vi "Main.vi"() -> ()   [LabVIEW 2019]
uses:
  Controls/States.ctl
  <vilib>/Gustavo Trejo/PIC Serial Toolkit/Controls/TRISA.ctl
  <vilib>/Gustavo Trejo/PIC Serial Toolkit/Controls/TRISB.ctl
  <vilib>/Gustavo Trejo/PIC Serial Toolkit/Controls/TRISC.ctl
  <vilib>/Gustavo Trejo/PIC Serial Toolkit/Controls/TRISD.ctl
  <vilib>/Gustavo Trejo/PIC Serial Toolkit/Controls/TRISE.ctl
  <vilib>/Gustavo Trejo/PIC Serial Toolkit/Controls/Pin Number.ctl
panel:
  out "Down":bool
  out "Up":bool
  in  "COM":refnum<visa-resource-name>
  out "Estado":string
  in  "Stop":bool
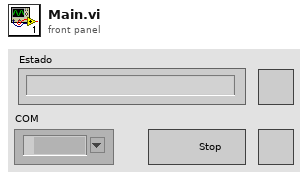
[diagram p1: front panel]
types:
  T1 = typedef "TRISE.ctl" = cluster{"E0":bool, "E1":bool, "E2":bool}
  T2 = typedef "TRISD.ctl" = cluster{"D0":bool, "D1":bool, "D2":bool, "D3":bool, "D4":bool, "D5":bool, "D6":bool, "D7":bool}
  T3 = typedef "TRISC.ctl" = cluster{"C0":bool, "C1":bool, "C2":bool, "C3":bool, "C4":bool, "C5":bool}
  T4 = typedef "TRISB.ctl" = cluster{"B0":bool, "B1":bool, "B2":bool, "B3":bool, "B4":bool, "B5":bool, "B6":bool, "B7":bool}
  T5 = typedef "TRISA.ctl" = cluster{"A0":bool, "A1":bool, "A2":bool, "A3":bool, "A4":bool, "A5":bool, "A6":bool, "A7":bool}
  T6 = typedef "States.ctl" = enum16{"Start", "GoDown", "BeDown", "GoUp", "BeUp", "Error", "Finish"}
  T7 = typedef "Pin Number.ctl" = enum16{"A0/AN0", "A1/AN1", "A2/AN2", "A3/AN3", "A4", "A5/AN4", "A6", "A7", "B0/AN12", "B1/AN10", "B2/AN8", "B3/AN9", "B4/AN11", "B5/AN13", "B6", "B7", "C0", "C1/PWM2", "C2/PWM1", "C3", "C4", "C5", "D0", "D1", "D2", "D3", "D4", "D5", "D6", "D7", "E0/AN5", "E1/AN6", "E2/AN7"}
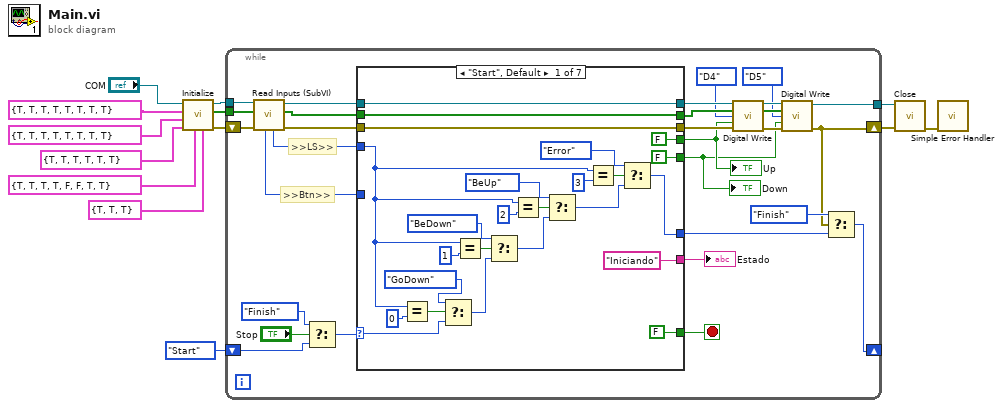
[diagram p0: block diagram]
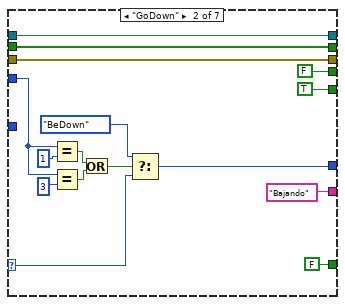
[diagram p2: hidden frame]
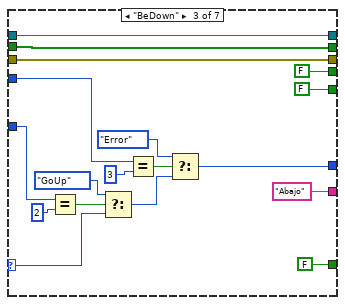
[diagram p3: hidden frame]
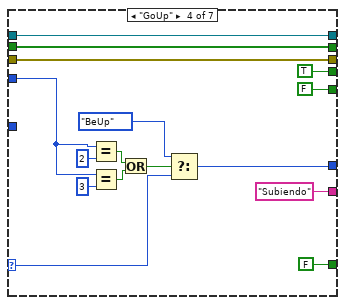
[diagram p4: hidden frame]
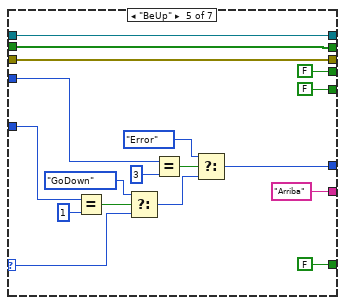
[diagram p5: hidden frame]
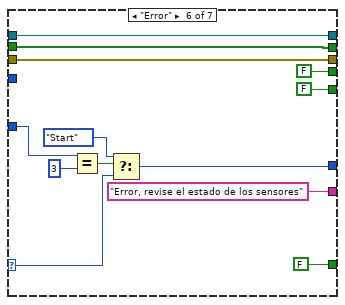
[diagram p6: hidden frame]
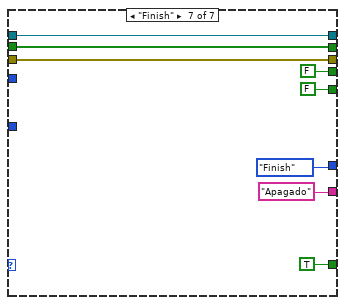
[diagram p7: hidden frame]
diagram:
  n1 = call <vilib>:"Initialize.vi"("TRISE E0-E2"=T1 {"E0"=TRUE, "E1"=TRUE, "E2"=TRUE}, "TRISD D0-D7"=T2 {"D0"=TRUE, "D1"=TRUE, "D2"=TRUE, "D3"=TRUE, "D4"=FALSE, "D5"=FALSE, "D6"=TRUE, "D7"=TRUE}, "TRISC C0-C5"=T3 {"C0"=TRUE, "C1"=TRUE, "C2"=TRUE, "C3"=TRUE, "C4"=TRUE, "C5"=TRUE}, "TRISB B0-B7"=T4 {"B0"=TRUE, "B1"=TRUE, "B2"=TRUE, "B3"=TRUE, "B4"=TRUE, "B5"=TRUE, "B6"=TRUE, "B7"=TRUE}, "TRISA A0-A7"=T5 {"A0"=TRUE, "A1"=TRUE, "A2"=TRUE, "A3"=TRUE, "A4"=TRUE, "A5"=TRUE, "A6"=TRUE, "A7"=TRUE}, "VISA Refnum in"="COM") -> ("error out"=w12:errorcluster, "Ports Ref Out"=w5:bool[], "VISA Refnum out"=w4:refnum<visa-resource-name>)  [unwired: 3 in]
  n2 = while {
    shift-right: [w36] -> _
    shift-left: States."Start" -> [w39]
    shift-right: [w16] -> w3
    shift-left: w12 -> [w33]
    tunnel: w5 -> [w31]
    tunnel: w4 -> [w30]
    tunnel: [w17] -> w2
    stop <- w38 stop-if-true
    # ">>LS>>"
    # ">>Btn>>"
    n3 = call "Read Inputs (SubVI).vi"("error in (no error)"=w33, "Ports Ref In"=w31, "VISA Refnum in"=w30) -> ("error out"=w32:errorcluster, "Ports Ref Out"=w26:bool[], "VISA Refnum out"=w27:refnum<visa-resource-name>, "LS"=w29:u32, "Btn"=w28:u32)  [unwired: 4 in]
    n4 = Select(t=States."Finish", s="Stop", f=w39) -> (s? t:f=w40:T6)
    n5 = case shown="\"Start\", Default" w40 {
      selector: w40 -> [w50 w77 w99 w103 w119 w137 _]
      tunnel: [FALSE FALSE FALSE FALSE FALSE FALSE TRUE] -> w38
      tunnel: [w66 w74 w90 w109 w125 w144 w154] -> w23
      tunnel: w32 -> [w66 w74 w90 w109 w125 w144 w154]
      tunnel: w29 -> [w52 w81 w96 w111 w127 _ _]
      tunnel: w28 -> [_ _ w101 _ w128 w148 _]
      tunnel: [w51 w75 w91 w110 w126 w138 States."Finish"] -> w35
      tunnel: ["Iniciando" "Bajando" "Abajo" "Subiendo" "Arriba" "Error, revise el estado de los sensores" "Apagado"] -> w34
      tunnel: [FALSE ("Abajo") TRUE ("Abajo") FALSE ("Abajo") FALSE ("Abajo") FALSE ("Abajo") FALSE ("Abajo") FALSE ("Abajo")] -> w14
      tunnel: [FALSE ("Arriba") FALSE ("Arriba") FALSE ("Arriba") TRUE ("Arriba") FALSE ("Arriba") FALSE ("Arriba") FALSE ("Arriba")] -> w15
      tunnel: [w44 w69 w85 w104 w120 w139 w150] -> w25
      tunnel: w27 -> [w44 w69 w85 w104 w120 w139 w150]
      tunnel: [w43 w68 w84 w102 w118 w136 w149] -> w24
      tunnel: w26 -> [w43 w68 w84 w102 w118 w136 w149]
      frame "Start", Default {
        n6 = Equal?(x=w52, y=u32 0) -> (x = y?=w63:bool)
        n7 = Select(t=States."GoDown", s=w63, f=w50) -> (s? t:f=w48:T6)
        n8 = Equal?(x=w52, y=u32 1) -> (x = y?=w62:bool)
        n9 = Select(t=States."BeDown", s=w62, f=w48) -> (s? t:f=w57:T6)
        n10 = Equal?(x=w52, y=u32 2) -> (x = y?=w59:bool)
        n11 = Select(t=States."BeUp", s=w59, f=w57) -> (s? t:f=w54:T6)
        n12 = Equal?(x=w52, y=u32 3) -> (x = y?=w56:bool)
        n13 = Select(t=States."Error", s=w56, f=w54) -> (s? t:f=w51:T6)
      }
      frame "GoDown" {
        n14 = Equal?(x=w81, y=u32 1) -> (x = y?=w83:bool)
        n15 = Equal?(x=w81, y=u32 3) -> (x = y?=w82:bool)
        n16 = Or(x=w83, y=w82) -> (x .or. y?=w78:bool)
        n17 = Select(t=States."BeDown", s=w78, f=w77) -> (s? t:f=w75:T6)
      }
      frame "BeDown" {
        n18 = Equal?(x=w101, y=u32 2) -> (x = y?=w98:bool)
        n19 = Select(t=States."GoUp", s=w98, f=w99) -> (s? t:f=w94:T6)
        n20 = Equal?(x=w96, y=u32 3) -> (x = y?=w93:bool)
        n21 = Select(t=States."Error", s=w93, f=w94) -> (s? t:f=w91:T6)
      }
      frame "GoUp" {
        n22 = Equal?(x=w111, y=u32 2) -> (x = y?=w117:bool)
        n23 = Equal?(x=w111, y=u32 3) -> (x = y?=w116:bool)
        n24 = Or(x=w117, y=w116) -> (x .or. y?=w115:bool)
        n25 = Select(t=States."BeUp", s=w115, f=w103) -> (s? t:f=w110:T6)
      }
      frame "BeUp" {
        n26 = Equal?(x=w128, y=u32 1) -> (x = y?=w135:bool)
        n27 = Select(t=States."GoDown", s=w135, f=w119) -> (s? t:f=w134:T6)
        n28 = Equal?(x=w127, y=u32 3) -> (x = y?=w133:bool)
        n29 = Select(t=States."Error", s=w133, f=w134) -> (s? t:f=w126:T6)
      }
      frame "Error" {
        n30 = Equal?(x=w148, y=u32 3) -> (x = y?=w146:bool)
        n31 = Select(t=States."Start", s=w146, f=w137) -> (s? t:f=w138:T6)
      }
      frame "Finish" {
      }
    }
    "Estado" <- w34
    "Up" <- w15
    "Down" <- w14
    n32 = call <vilib>:"Digital Write.vi"("VISA Refnum in"=w25, "Ports Ref In"=w24, "Pin Number"=Pin_Number."D4", "State Output"=w15, "error in (no error)"=w23) -> ("VISA Refnum out"=w21:refnum<visa-resource-name>, "Ports Ref Out"=w20:bool[], "error out"=w19:errorcluster)  [unwired: 8 in]
    n33 = call <vilib>:"Digital Write.vi"("VISA Refnum in"=w21, "Ports Ref In"=w20, "Pin Number"=Pin_Number."D5", "State Output"=w14, "error in (no error)"=w19) -> ("VISA Refnum out"=w17:refnum<visa-resource-name>, "error out"=w16:errorcluster)  [unwired: 8 in, 1 out]
    n34 = Select(t=States."Finish", s=w16, f=w35) -> (s? t:f=w36:T6)
  }
  n35 = call <vilib>:"Close.vi"("error in (no error)"=w3, "VISA Refnum in"=w2) -> ("error out"=w1:errorcluster)  [unwired: 9 in]
  n36 = call <vilib>:"Simple Error Handler.vi"("error in (no error)"=w1) -> ()  [unwired: 4 in, 5 out]
